vi "LM model function and gradient (IRF deconvolution + 1-Exp).vi"(3 "output control":T1, 4 "data":variant, 5 "X":dbl[](array[numeric]), 6 "a":dbl[](array[numeric])) -> (0 "error out":errorcluster, 1 "f'(X,a)":dbl[][](array[numeric]), 2 "f(X,a)":dbl[](array[numeric]))   [LabVIEW 2021, in "Fits.lvlib"]
doc: "This template is the starting point for creating a model function to be passed to the Nonlinear Curve Fit.vi."
uses:
  Fits.lvlib
  <vilib>/Analysis/NI_AALPro.lvlib
  IRF Deconvolution Parameters.ctl
  <vilib>/Analysis/2dsp.llb/1D Convolution (DBL).vi
  Arrays/Arrays.lvlib
  ded07d26-2b4e-4479-8624-e9e472b16fe6.vi
  <vilib>/gmath/NumericalOptimization/LM_output select.ctl
  <vilib>/gmath/NI_Gmath.lvlib
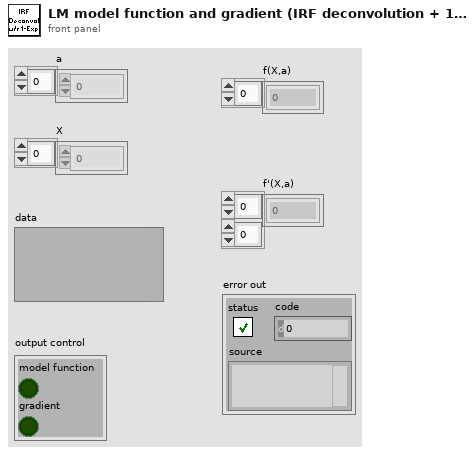
[diagram p1: front panel]
types:
  T1 = typedef "NI_Gmath.lvlib/LM_output select.ctl" = cluster{"model function":bool, "gradient":bool}
  T2 = typedef "Fits.lvlib/IRF Deconvolution Parameters.ctl" = cluster{"IRF support":dbl[], "Lifetime":dbl}
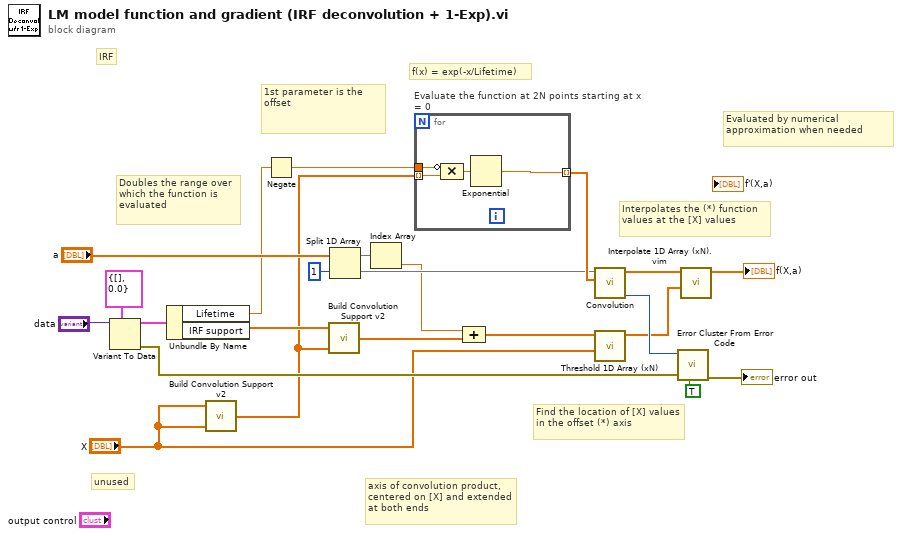
[diagram p0: block diagram]
diagram:
  # "1st parameter is the offset"
  # "Doubles the range over which the function is evaluated"
  # "unused"
  # "Evaluated by numerical approximation when needed"
  # "Interpolates the (*) function values at the [X] values"
  # "Find the location of [X] values in the offset (*) axis"
  # "axis of convolution product, centered on [X] and extended at both ends"
  # "f(x) = exp(-x/Lifetime)"
  # "IRF"
  n1 = Variant To Data(type=T2 {"IRF support"=[], "Lifetime"=0.0} ("IRF"), Variant="data") -> (data=w20:T2, error out=w14:errorcluster)  [unwired: 1 in]
  n2 = Unbundle By Name(w20) -> ("Lifetime"=w6:dbl, "IRF support"=w13:dbl[])
  n3 = call "Build Convolution Support v2.vi"("X Array 2"="X", "X Array 1"="X") -> ("X Arrays Convolution Support"=w8:dbl[])  [unwired: 3 in]
  n4 = Negate(x=w6) -> (-x=w7:dbl)
  n5 = call "Build Convolution Support v2.vi"("X Array 2"=w8, "X Array 1"=w13) -> ("X Arrays Convolution Support"=w12:dbl[])  [unwired: 3 in]
  n6 = Split 1D Array(array="a", index=1) -> (first subarray=w2:dbl[], second subarray=w3:dbl[])
  n7 = Index Array(array=w2) -> (element=w1:dbl)  [unwired: 1 in]
  n8 = for "Evaluate the function at 2N points starting at x = 0" {
    tunnel: [w24] -> w19 mode=indexing
    tunnel: w8 -> [w26] mode=indexing
    tunnel: w7 -> [w25]
    n9 = Compound Arithmetic op=MULTIPLY(invert w25, w26) -> (w27:dbl)
    n10 = Exponential(1:w27) -> (0:w24:dbl)
  }
  n11 = Compound Arithmetic op=ADD(w1, w12) -> (w5:dbl[])
  n12 = call-poly <vilib>:"Convolution.vi"("Y"=w19, "X"=w3) -> ("error"=w18:i32, "X * Y"=w11:dbl[])  [unwired: 8 in]
  n13 = call "Threshold 1D Array (xN).vi"("Search Values"="X", "X"=w5) -> ("Interpolated Indices"=w15:dbl[])  [unwired: 9 in]
  n14 = call <vilib>:"Error Cluster From Error Code.vi"("show call chain? (False)"=TRUE, "error in (no error)"=w14, "error code (0)"=w18) -> ("error out"=→"error out":errorcluster)  [unwired: 6 in]
  n15 = call "Interpolate 1D Array (xN).vim"("Interpolated Indices"=w15, "Y"=w11) -> ("Interpolated Y"=→"f(X,a)":dbl[])  [unwired: 9 in]
